vi "wmf_open_camera.vi"(8 "error in (no error)":errorcluster, 10 "Config path":path, 11 "camera_name":string) -> (0 "error out":errorcluster, 2 "height":i32, 3 "width":i32)   [LabVIEW 2024, in "Vision.lvlib"]
uses:
  Vision.lvlib
  <vilib>/Utility/config.llb/Read Key (I32).vi
  <vilib>/Utility/config.llb/Read Key (String).vi
  <vilib>/Utility/config.llb/NI_LVConfig.lvlib
  bin/LVWMF.dll
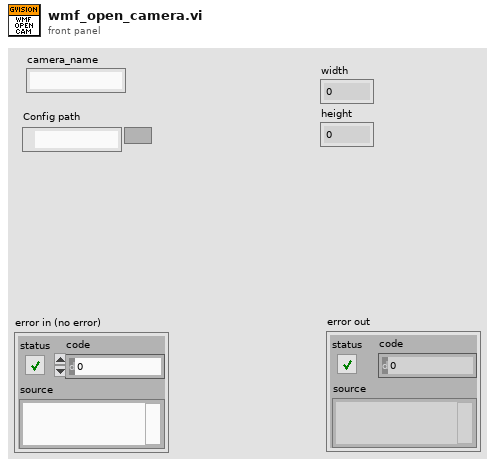
[diagram p1: front panel]
types:
  T1 = typedef "NI_LVConfig.lvlib/Config Data RefNum.ctl" = refnum<k1>
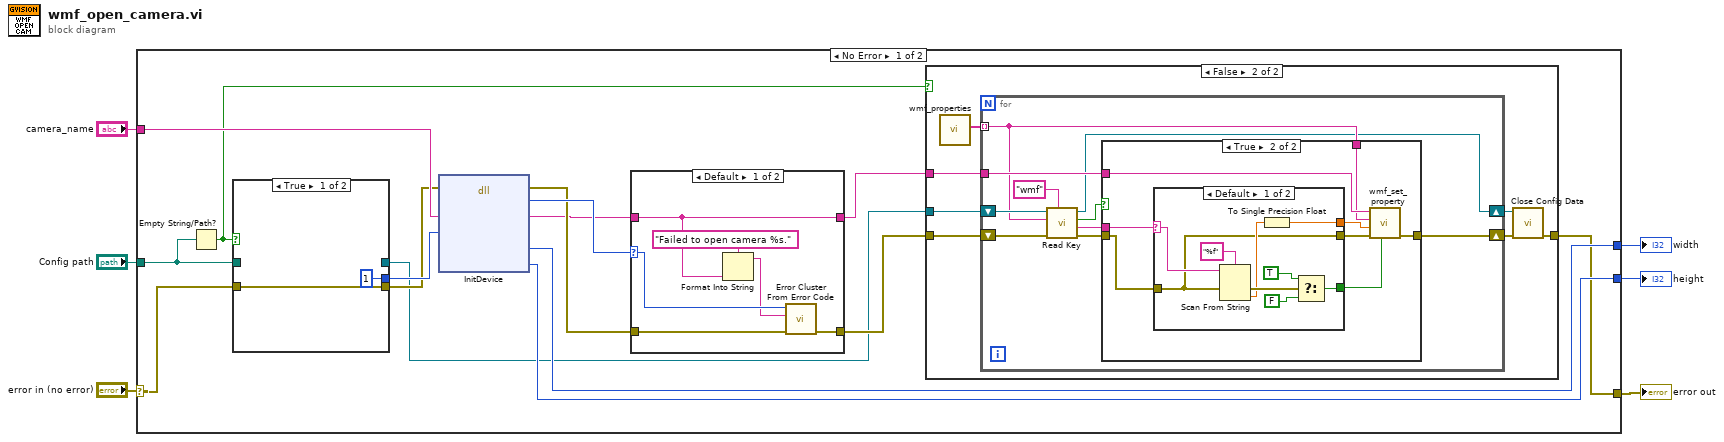
[diagram p0: block diagram]
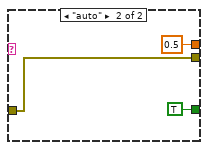
[diagram p4: hidden frame]
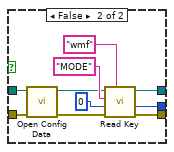
[diagram p5: hidden frame]
diagram:
  n1 = case shown="No Error" "error in (no error)" {
    selector: "error in (no error)" -> [w19 w81]
    tunnel: [w9 w81] -> w4
    tunnel: "camera_name" -> [w18 _]
    tunnel: "Config path" -> [w8 _]
    tunnel: [w17 _] -> w2
    tunnel: [w16 _] -> w1
    frame No Error {
      n2 = Empty String/Path?(string/path=w8) -> (empty?=w7:bool)
      n3 = case shown="True" w7 {
        tunnel: w19 -> [w62 w72]
        tunnel: [1 ("value") w67] -> w15
        tunnel: [w62 w66] -> w14
        tunnel: [_ w64] -> w10
        tunnel: w8 -> [_ w63]
        frame True {
        }
        frame False {
          n4 = call <vilib>:"Open Config Data.vi"("error in (no error)"=w72, "configuration file path"=w63) -> ("error out"=w65:errorcluster, "refnum"=w68:T1)  [unwired: 7 in, 1 out]
          n5 = call-poly <vilib>:"Read Key.vi"("section"="wmf", "error in (no error)"=w65, "default value"=0, "key"="MODE", "refnum"=w68) -> ("error out"=w66:errorcluster, "value"=w67:i32, "refnum out"=w64:T1)  [unwired: 3 in, 1 out]
        }
      }
      n6 = dll-call lib="C:/Users/cfang/Desktop/nebraska-silicon-lab/pixel-gantry-control/Gantry/Shared Components/bin/LVWMF.dll" fn="InitDevice"(error in=w14, "camera_name"=w18, "mode_id"=w15) -> (error out=w20:errorcluster, "return type"=w21:i32, "camera_name"=w13:string, "width"=w17:i32, "height"=w16:i32)  [unwired: 5 in, 1 out]
      n7 = case shown="Default" w21 {
        selector: w21 -> [w76 _]
        tunnel: w20 -> [w78 w80]
        tunnel: [w77 w80] -> w12
        tunnel: w13 -> [w73 w79]
        tunnel: [w73 w79] -> w11
        frame Default {
          n8 = Format Into String(format string="Failed to open camera %s." ("error message (\"\")"), w73) -> (resulting string=w74:string)  [unwired: 2 in, 1 out]
          n9 = call <vilib>:"Error Cluster From Error Code.vi"("error in (no error)"=w78, "error message (\"\")"=w74, "error code (0)"=w76) -> ("error out"=w77:errorcluster)  [unwired: 6 in]
        }
        frame 0 {
        }
      }
      n10 = case shown="False" w7 {
        tunnel: w12 -> [w22 w29]
        tunnel: w11 -> [_ w28]
        tunnel: w10 -> [_ w27]
        tunnel: [w22 w24] -> w9
        frame True {
        }
        frame False {
          n11 = call "wmf_properties.vi"() -> ("WMF Properties"=w23:string[])  [unwired: 11 in]
          n12 = for {
            tunnel: w23 -> [w32] mode=indexing
            shift-right: [w31] -> w26
            shift-left: w27 -> [w39]
            shift-right: [w34] -> w25
            shift-left: w29 -> [w37]
            tunnel: w28 -> [w33]
            n13 = call-poly <vilib>:"Read Key.vi"("section"="wmf", "error in (no error)"=w37, "key"=w32, "refnum"=w39) -> ("error out"=w35:errorcluster, "value"=w36:string, "found?"=w30:bool, "refnum out"=w31:T1)  [unwired: 4 in]
            n14 = case shown="True" w30 {
              tunnel: w36 -> [_ w48]
              tunnel: w35 -> [w40 w47]
              tunnel: [w40 w45] -> w34
              tunnel: w33 -> [_ w44]
              tunnel: w32 -> [_ w43]
              frame False {
              }
              frame True {
                n15 = case shown="Default" w48 {
                  selector: w48 -> [w57 _]
                  tunnel: [w52 TRUE] -> w41
                  tunnel: [w55 sgl 0.5] -> w42
                  tunnel: w47 -> [w51 w60]
                  tunnel: [w51 w60] -> w46
                  frame Default {
                    n16 = Scan From String(format string="%f", input string=w57, error in=w51) -> (error out=w54:errorcluster, output 1=w53:dbl)  [unwired: 2 in, 2 out]
                    n17 = To Single Precision Float(number=w53) -> (single precision float=w55:sgl)
                    n18 = Select(t=TRUE, s=w54, f=FALSE) -> (s? t:f=w52:bool)
                  }
                  frame "auto" {
                  }
                }
                n19 = call "wmf_set_property.vi"("Auto"=w41, "error in (no error)"=w46, "Value"=w42, "property name"=w43, "camera_name"=w44) -> ("error out"=w45:errorcluster)  [unwired: 6 in]
              }
            }
          }
          n20 = call <vilib>:"Close Config Data.vi"("error in (no error)"=w25, "refnum"=w26) -> ("error out"=w24:errorcluster)  [unwired: 8 in, 1 out]
        }
      }
    }
    frame Error {
    }
  }
  "error out" <- w4
  "width" <- w2
  "height" <- w1
